vi "DataLog Databases_srv.vi"(7 "certificate in":string) -> (8 "database names":string[](array[string]), 15 "error out":errorcluster)   [LabVIEW 2012]
uses:
  clientsrv/typedefs/t_ClientSrv Access Levels.ctl
  typedefs/t_DataLog Databases Methods.ctl
panel:
  # "Update panel typedef\nafter changing panel."
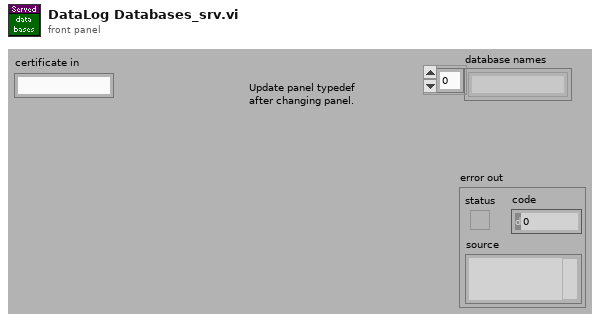
[diagram p1: front panel]
types:
  T1 = typedef "t_DataLog Databases Methods.ctl" = enum16{"initialize", "get ref", "get names", "cleanup"}
  T2 = typedef "t_ClientSrv Access Levels.ctl" = enum16{"observer", "operator", "local"}
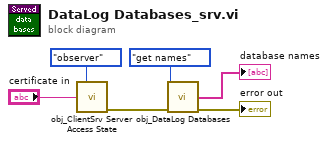
[diagram p0: block diagram]
diagram:
  n1 = call "obj_ClientSrv Server Access State.vi"("access level"=t_ClientSrv_Access_Levels."observer", "certificate in"="certificate in") -> ("error out"=w6:errorcluster)  [unwired: 11 in, 2 out]
  n2 = call "obj_DataLog Databases.vi"("method"=t_DataLog_Databases_Methods."get names", "error in (no error)"=w6) -> ("database names"=→"database names":string[], "error out"=→"error out":errorcluster)  [unwired: 11 in, 1 out]
